vi "RP100.Set Output State.vi"(8 "error in (no error)":errorcluster, 9 "Output State":T2=enum."Enabled", 10 "Output Channel":T1, 11 "VISA resource name":refnum<visa-resource-name>) -> (0 "error out":errorcluster, 2 "Output Channel":T1, 3 "VISA Refnum out":refnum<visa-resource-name>)   [LabVIEW 2019, in "Inst.RP100.lvclass"]
uses:
  Inst.RP100.lvclass
  Typedefs/Output Channel--Enum.ctl
  Typedefs/Output State--Enum.ctl
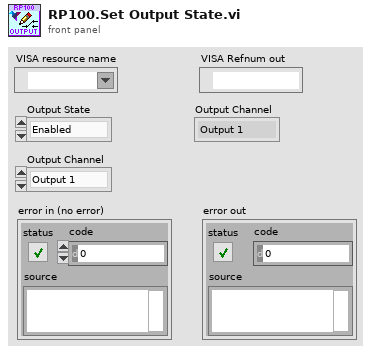
[diagram p1: front panel]
types:
  T1 = typedef "Inst.RP100.lvclass/Output Channel--Enum.ctl" = enum16{"Output 1", "Output 2"}
  T2 = typedef "Inst.RP100.lvclass/Output State--Enum.ctl" = enum16{"Shorted", "Enabled"}
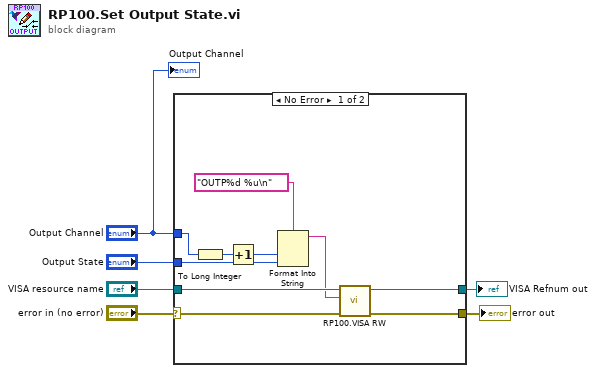
[diagram p0: block diagram]
diagram:
  n1 = case shown="No Error" "error in (no error)" {
    selector: "error in (no error)" -> [w11 w18]
    tunnel: "VISA resource name" -> [w13 w17]
    tunnel: [w10 w18] -> w5
    tunnel: [w9 w17] -> w4
    tunnel: "Output Channel" -> [w16 _]
    tunnel: "Output State" -> [w14 _]
    frame No Error {
      n2 = To Long Integer(number=w16) -> (32bit integer=w8:i32)
      n3 = Increment(x=w8) -> (x+1=w7:i32)
      n4 = Format Into String(format string="OUTP%d %u\n", w7, w14) -> (resulting string=w12:string)  [unwired: 2 in, 1 out]
      n5 = call "RP100.VISA RW.vi"("error in (no error)"=w11, "Write"=w12, "VISA Refnum in"=w13) -> ("error out"=w10:errorcluster, "VISA Refnum out"=w9:refnum<visa-resource-name>)  [unwired: 6 in, 1 out]
    }
    frame Error {
    }
  }
  "VISA Refnum out" <- w4
  "error out" <- w5
  "Output Channel" <- "Output Channel"
